vi "BuildScript.vi"() -> ()   [LabVIEW 2014]
uses:
  Bus.lvclass
panel:
  out "ErrorArray":errorcluster[](array[cluster])
  in  "ErrorArray":errorcluster[](array[cluster])
  out "Script":string[](array[string])
  out "Bus":refnum<class "Bus.lvclass">
  in  "Bus":refnum<class "Bus.lvclass">
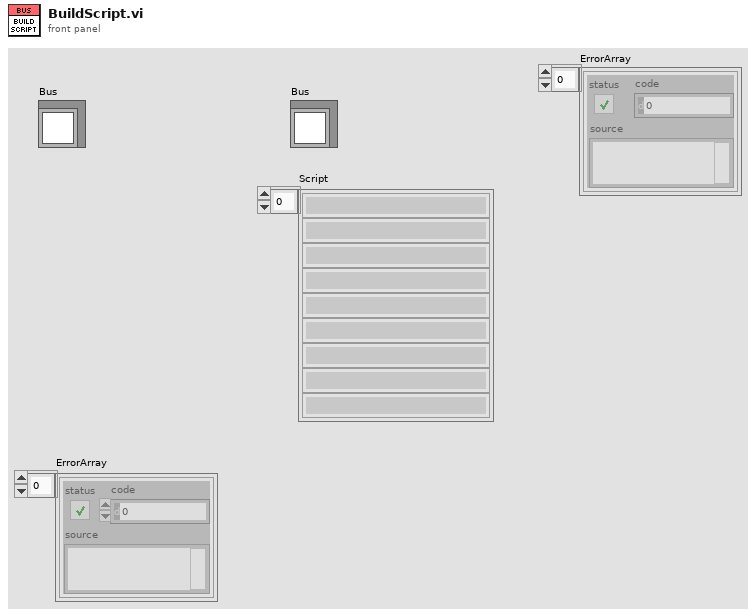
[diagram p1: front panel]
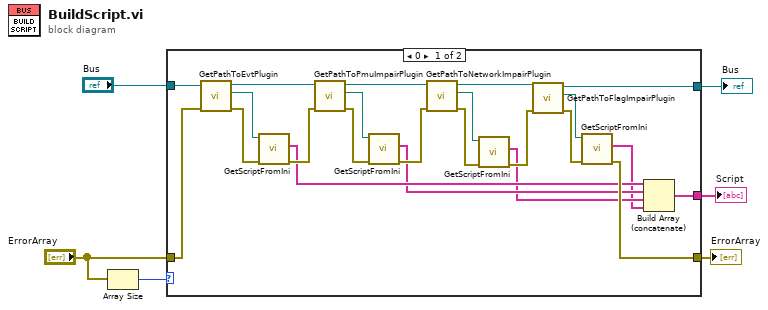
[diagram p0: block diagram]
diagram:
  n1 = Array Size(array="ErrorArray") -> (size(s)=w6:i32)
  n2 = case shown="0" w6 {
    tunnel: "ErrorArray" -> [w29 w31]
    tunnel: "Bus" -> [w28 w30]
    tunnel: [w14 w31] -> w3
    tunnel: [w12 w30] -> w2
    tunnel: [w7 _] -> w1
    frame 0 {
      n3 = call "GetPathToEvtPlugin.vi"("ErrorArray In"=w29, "Bus.lvclass In"=w28) -> ("ErrorArray Out"=w26:errorcluster[], "EvtPluginINIFilePath"=w27:path, "Bus.lvclass Out"=w25:refnum<class "Bus.lvclass">)  [unwired: 7 in]
      n4 = call "GetScriptFromIni.vi"("ErrorArray"=w26, "PathtoIniFile"=w27) -> ("ErrorArray"=w24:errorcluster[], "Script"=w11:string[])  [unwired: 8 in]
      n5 = call "GetPathToPmuImpairPlugin.vi"("ErrorArray In"=w24, "Bus.lvclass In"=w25) -> ("ErrorArray Out"=w22:errorcluster[], "PmuImpairPluginINIFilePath"=w23:path, "Bus.lvclass Out"=w21:refnum<class "Bus.lvclass">)  [unwired: 7 in]
      n6 = call "GetScriptFromIni.vi"("ErrorArray"=w22, "PathtoIniFile"=w23) -> ("ErrorArray"=w20:errorcluster[], "Script"=w10:string[])  [unwired: 8 in]
      n7 = call "GetPathToNetworkImpairPlugin.vi"("ErrorArray In"=w20, "Bus.lvclass In"=w21) -> ("ErrorArray Out"=w19:errorcluster[], "NetImpPluginINIFilePath"=w18:path, "Bus.lvclass Out"=w16:refnum<class "Bus.lvclass">)  [unwired: 7 in]
      n8 = call "GetScriptFromIni.vi"("ErrorArray"=w19, "PathtoIniFile"=w18) -> ("ErrorArray"=w17:errorcluster[], "Script"=w9:string[])  [unwired: 8 in]
      n9 = call "GetPathToFlagImpairPlugin.vi"("ErrorArray In"=w17, "Bus.lvclass In"=w16) -> ("ErrorArray Out"=w15:errorcluster[], "FlagImpPluginINIFilePath"=w13:path, "Bus.lvclass Out"=w12:refnum<class "Bus.lvclass">)  [unwired: 7 in]
      n10 = call "GetScriptFromIni.vi"("ErrorArray"=w15, "PathtoIniFile"=w13) -> ("ErrorArray"=w14:errorcluster[], "Script"=w8:string[])  [unwired: 8 in]
      n11 = Build Array (concatenate)(w11, w10, w9, w8) -> (w7:string[])
    }
    frame 1, Default {
    }
  }
  "Bus" <- w2
  "Script" <- w1
  "ErrorArray" <- w3
